vi "AxisSteps.vi"() -> ()   [LabVIEW 2011]
panel:
  in  "Stack_Steps":dbl
  in  "Slow_Axis_Steps":dbl
  in  "Fast_Axis_Steps":dbl
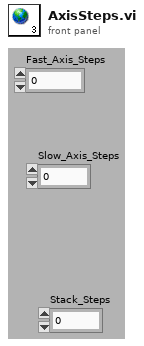
[diagram p1: front panel]
diagram:
